vi "Parse Comments from CtlExp.vi"(7 "error in":errorcluster, 10 "ENTIRE Array of YAML Lines":string[](array[string])) -> (0 "error out":errorcluster, 1 "device details":string[][](array[string]), 2 "lockin contents":string[][](array[string]), 3 "wiring":string[][](array[string]))   [LabVIEW 2016]
uses:
  <userlib>/_OpenG.lib/dictionary/dictionary.llb/Dictionary Object RefNum__ogtk.ctl
  <userlib>/_OpenG.lib/dictionary/dictionary.llb/Dictionary Object RefNum - Enum__ogtk.ctl
panel:
  out "items":cluster{"key":variant, "value":variant}[](array[cluster])
  out "lockin stuff":string
  out "lockin contents":cluster{"key":variant, "value":variant}[](array[cluster])
  out "expt content":cluster{"key":variant, "value":variant}[](array[cluster])
  out "device contents":cluster{"key":variant, "value":variant}[](array[cluster])
  out "date":string
  out "Dictionary Items":cluster{"key":variant, "value":variant}[](array[cluster])
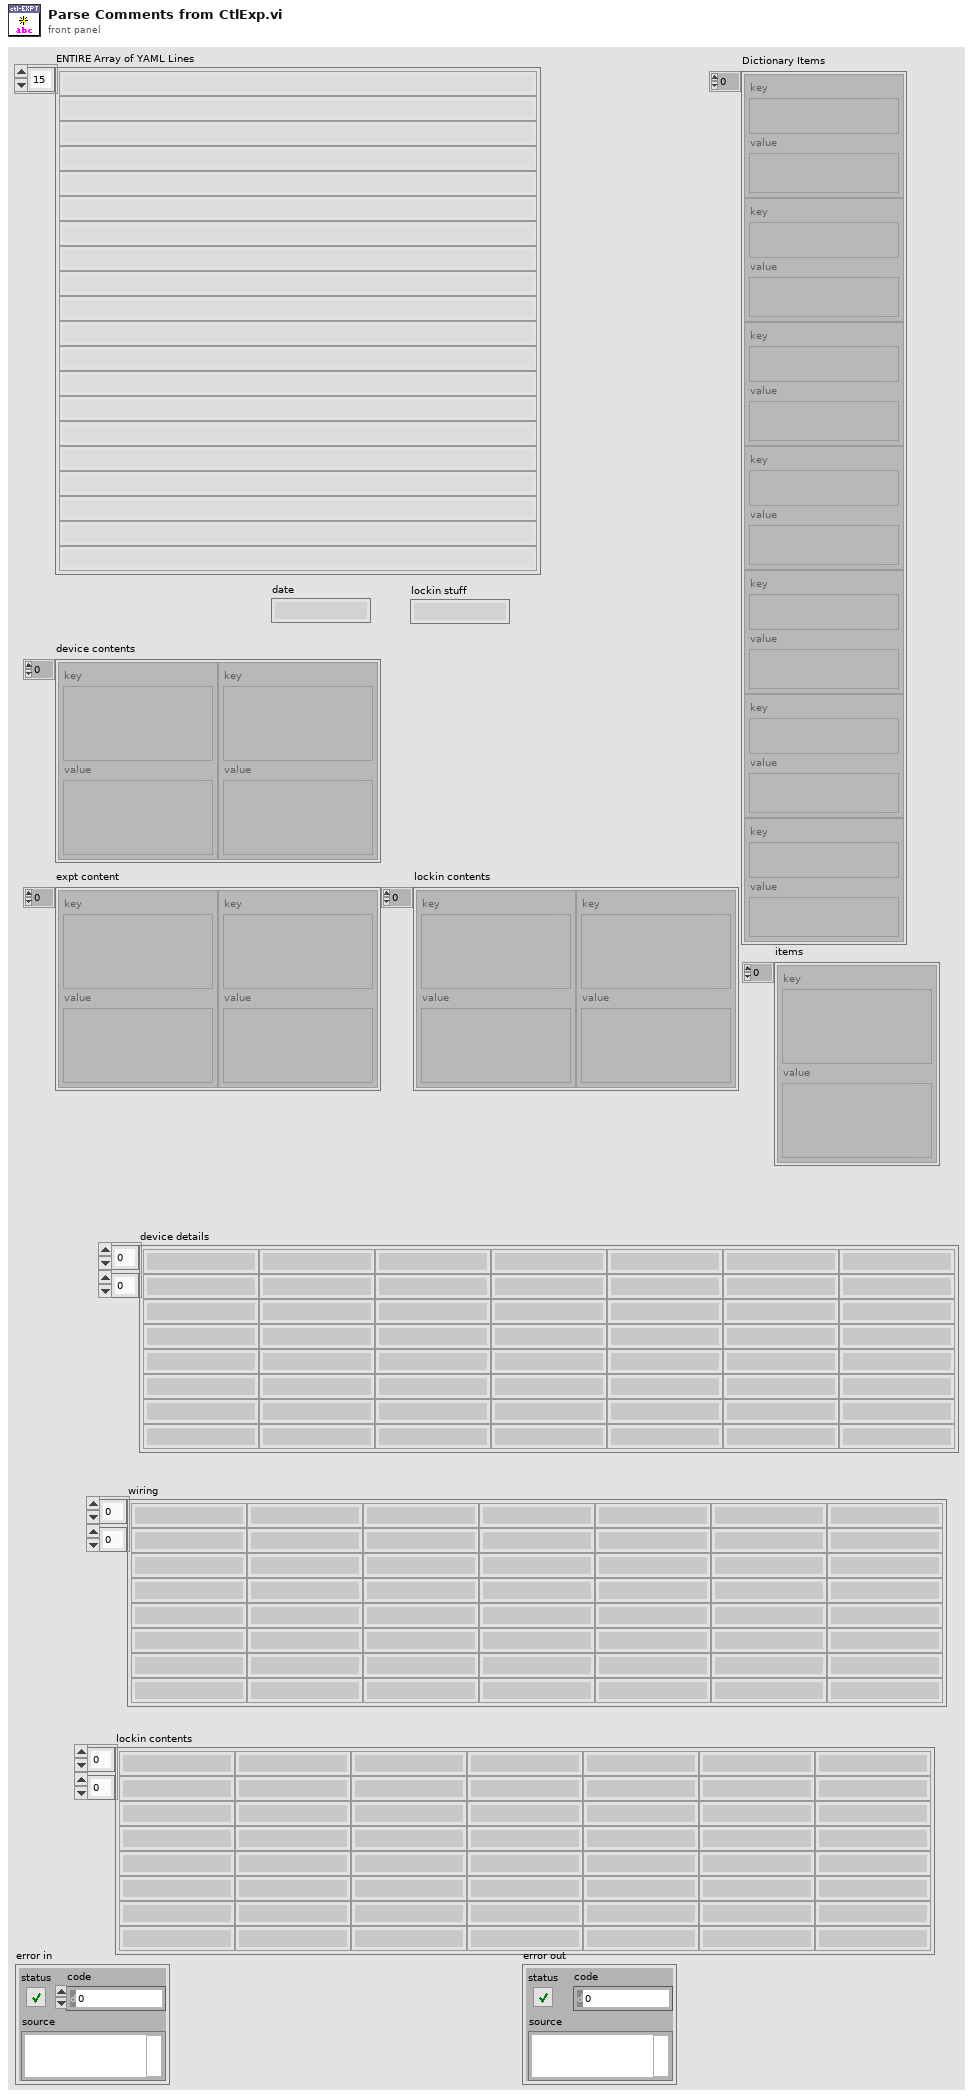
[diagram p1: front panel]
types:
  T1 = typedef "Dictionary Object RefNum__ogtk.ctl" = refnum<k1>
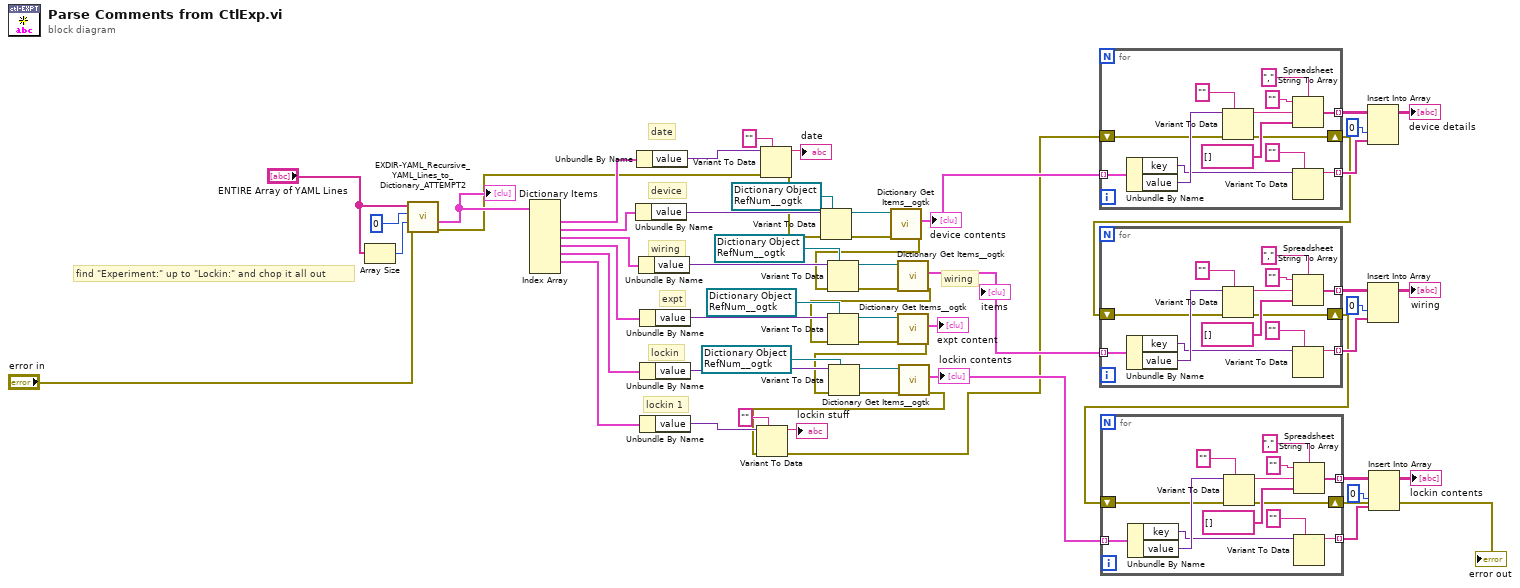
[diagram p0: block diagram]
diagram:
  w32 = T1 refnum items=["Dictionary"] ("dictionary out")
  w39 = T1 refnum items=["Dictionary"] ("dictionary out")
  w42 = T1 refnum items=["Dictionary"] ("dictionary out")
  w46 = T1 refnum items=["Dictionary"] ("dictionary out")
  # "find \"Experiment:\" up to \"Lockin:\" and chop it all out"
  # "wiring"
  # "lockin 1"
  # "lockin"
  # "expt"
  # "wiring"
  # "device"
  # "date"
  n1 = Array Size(array="ENTIRE Array of YAML Lines") -> (size(s)=w58:i32)
  n2 = call "EXDIR-YAML_Recursive_YAML_Lines_to_Dictionary_ATTEMPT2.vi"("error in"="error in", "End Index"=w58, "Start Index"=0, "ENTIRE Array of YAML Lines"="ENTIRE Array of YAML Lines") -> ("error out"=w7:errorcluster, "items"=w57:cluster{"key":variant, "value":variant}[])  [unwired: 5 in, 1 out]
  "Dictionary Items" <- w57
  n3 = Index Array(array=w57) -> (element #1=w56:cluster{"key":variant, "value":variant}, element #2=w55:cluster{"key":variant, "value":variant}, element #3=w54:cluster{"key":variant, "value":variant}, element #4=w53:cluster{"key":variant, "value":variant}, element #5=w52:cluster{"key":variant, "value":variant}, element #6=w51:cluster{"key":variant, "value":variant})  [unwired: 7 in, 1 out]
  n4 = Unbundle By Name(w55) -> ("value"=w47:variant)
  n5 = Unbundle By Name(w56) -> ("value"=w50:variant)
  n6 = Unbundle By Name(w54) -> ("value"=w43:variant)
  n7 = Unbundle By Name(w53) -> ("value"=w40:variant)
  n8 = Unbundle By Name(w52) -> ("value"=w33:variant)
  n9 = Unbundle By Name(w51) -> ("value"=w29:variant)
  n10 = Variant To Data(error in=w7, type="", Variant=w50) -> (data=→"date":string, error out=w8:errorcluster)
  n11 = Variant To Data(error in=w8, type=w46, Variant=w47) -> (data=w45:T1, error out=w36:errorcluster)
  n12 = call <userlib>:"Dictionary Get Items__ogtk.vi"("error in (no error)"=w36, "dictionary"=w45) -> ("error out"=w11:errorcluster, "items"=w17:cluster{"key":variant, "value":variant}[])  [unwired: 7 in, 1 out]
  "device contents" <- w17
  n13 = Variant To Data(error in=w11, type=w42, Variant=w43) -> (data=w44:T1, error out=w37:errorcluster)
  n14 = call <userlib>:"Dictionary Get Items__ogtk.vi"("error in (no error)"=w37, "dictionary"=w44) -> ("error out"=w9:errorcluster, "items"=w28:cluster{"key":variant, "value":variant}[])  [unwired: 7 in, 1 out]
  "items" <- w28
  n15 = Variant To Data(error in=w9, type=w39, Variant=w40) -> (data=w41:T1, error out=w38:errorcluster)
  n16 = call <userlib>:"Dictionary Get Items__ogtk.vi"("error in (no error)"=w38, "dictionary"=w41) -> ("error out"=w10:errorcluster, "items"=→"expt content":cluster{"key":variant, "value":variant}[])  [unwired: 7 in, 1 out]
  n17 = Variant To Data(error in=w10, type=w32, Variant=w33) -> (data=w34:T1, error out=w35:errorcluster)
  n18 = call <userlib>:"Dictionary Get Items__ogtk.vi"("error in (no error)"=w35, "dictionary"=w34) -> ("error out"=w1:errorcluster, "items"=w12:cluster{"key":variant, "value":variant}[])  [unwired: 7 in, 1 out]
  "lockin contents" <- w12
  n19 = Variant To Data(error in=w1, type="", Variant=w29) -> (data=→"lockin stuff":string, error out=w2:errorcluster)
  n20 = for {
    tunnel: w17 -> [w72] mode=indexing
    tunnel: [w67] -> w20 mode=indexing
    tunnel: [w63] -> w18 mode=indexing
    shift-right: [w60] -> w5
    shift-left: w2 -> [w61]
    n21 = Unbundle By Name(w72) -> ("key"=w68:variant, "value"=w70:variant)
    n22 = Variant To Data(error in=w61, type="", Variant=w70) -> (data=w65:string, error out=w60:errorcluster)
    n23 = Spreadsheet String To Array(delimiter (Tab)=",", format string="", spreadsheet string=w65, array type (2D Dbl)=string[] []) -> (array=w63:string[])
    n24 = Variant To Data(type="", Variant=w68) -> (data=w67:string)  [unwired: 1 in, 1 out]
  }
  n25 = for {
    tunnel: w28 -> [w85] mode=indexing
    tunnel: [w80] -> w25 mode=indexing
    tunnel: [w76] -> w27 mode=indexing
    shift-right: [w73] -> w4
    shift-left: w5 -> [w74]
    n26 = Unbundle By Name(w85) -> ("key"=w81:variant, "value"=w83:variant)
    n27 = Variant To Data(error in=w74, type="", Variant=w83) -> (data=w78:string, error out=w73:errorcluster)
    n28 = Spreadsheet String To Array(delimiter (Tab)=",", format string="", spreadsheet string=w78, array type (2D Dbl)=string[] []) -> (array=w76:string[])
    n29 = Variant To Data(type="", Variant=w81) -> (data=w80:string)  [unwired: 1 in, 1 out]
  }
  n30 = for {
    tunnel: w12 -> [w98] mode=indexing
    tunnel: [w93] -> w15 mode=indexing
    tunnel: [w89] -> w13 mode=indexing
    shift-right: [w86] -> w3
    shift-left: w4 -> [w87]
    n31 = Unbundle By Name(w98) -> ("key"=w94:variant, "value"=w96:variant)
    n32 = Variant To Data(error in=w87, type="", Variant=w96) -> (data=w91:string, error out=w86:errorcluster)
    n33 = Spreadsheet String To Array(delimiter (Tab)=",", format string="", spreadsheet string=w91, array type (2D Dbl)=string[] []) -> (array=w89:string[])
    n34 = Variant To Data(type="", Variant=w94) -> (data=w93:string)  [unwired: 1 in, 1 out]
  }
  "error out" <- w3
  n35 = Insert Into Array(array=w18, index (col)=0 ("disabled index (col)"), new element=w20) -> (→"device details":string[][])  [unwired: 1 in]
  n36 = Insert Into Array(array=w27, index (col)=0 ("disabled index (col)"), new element=w25) -> (→"wiring":string[][])  [unwired: 1 in]
  n37 = Insert Into Array(array=w13, index (col)=0 ("disabled index (col)"), new element=w15) -> (→"lockin contents":string[][])  [unwired: 1 in]
